vi "PCSMain.get Objects PCS-wide.vi"(0 "i ref in":refnum<vi>, 5 "error in (no error)":errorcluster) -> (14 "i ref out":refnum<vi>, 19 "error out":errorcluster)   [LabVIEW 2014, in "PCSMain.lvlib"]
doc: "This VI gets certain objects running elsewhere in the PCS."
uses:
  PCSMain.lvlib
  CS_Core/CSSystem/CSSystemLib/CSSystemLib.lvlib
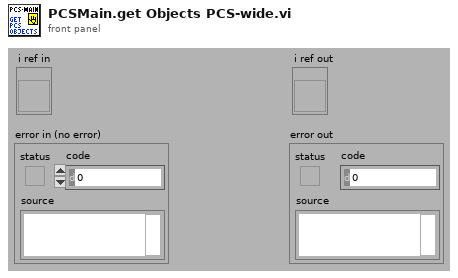
[diagram p1: front panel]
types:
  T1 = typedef "PCSMain.lvlib/PCSMain.i attribute.ctl" = cluster{"System Objects":cluster{"Spectrometer Objects":string[], "Camera Objects":string[], "Image Operator Objects":string[], "Gate- and Delaygenerators":string[], "Current Meas Objects":string[], "Calorimeter Objects":string[], "Powermeter Objects":string[], "SSAC Objects":string[], "Vacuum Control Objects":string[], "Countdown Counter Objects":string[], "Beckhoff Watchdog Objects":string[], "SHS Analyzer Objects":string[]}, "Local Objects":cluster{"Spectrometer Objects":string[], "Camera Objects":string[], "Image Operator Objects":string[], "Gate- and Delaygenerators":string[], "Current Meas Objects":string[], "Calorimeter Objects":string[], "Powermeter Objects":string[], "SSAC Objects":string[], "Vacuum Control Objects":string[], "Countdown Counter Objects":string[], "Beckhoff Watchdog Objects":string[], "SHS Analyzer Objects":string[]}, "Systems on same node":string[], "Data Viewer visible?":bool, "Running Objects":cluster{"Operators":bool, "SHS Analyzers":bool}, "Cam Instance System ID":string, "Black Box Objects":string[], "Switch Objects":string[], "Motion GUI Objects":string[], "Osci Objects":string[]}
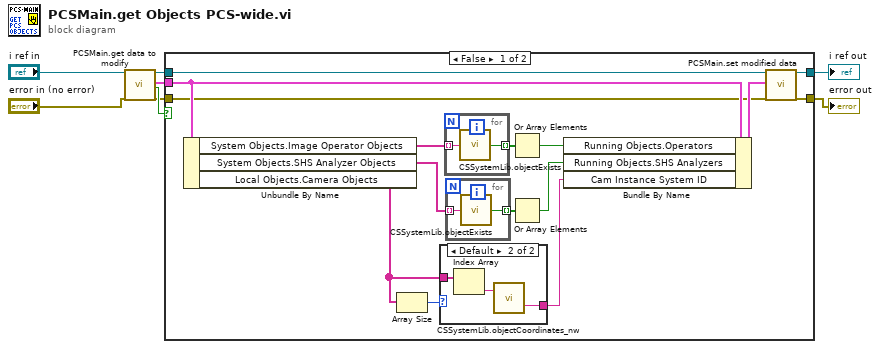
[diagram p0: block diagram]
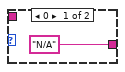
[diagram p2: hidden frame]
diagram:
  n1 = call "PCSMain.get data to modify.vi"("i ref in"="i ref in", "error in (no error)"="error in (no error)") -> ("i ref out"=w1:refnum<vi>, "i attribute"=w4:T1, "timed out"=w3:bool, "error out"=w2:errorcluster)  [unwired: 14 in]
  n2 = case shown="False" w3 {
    tunnel: w1 -> [w23 w33]
    tunnel: [w22 w33] -> w5
    tunnel: w2 -> [w18 w32]
    tunnel: [w21 w32] -> w6
    tunnel: w4 -> [w20 _]
    frame False {
      n3 = Unbundle By Name(w20) -> ("System Objects.Image Operator Objects"=w17:string[], "System Objects.SHS Analyzer Objects"=w14:string[], "Local Objects.Camera Objects"=w10:string[])
      n4 = Array Size(array=w10) -> (size(s)=w9:i32)
      n5 = case shown="Default" w9 {
        tunnel: w10 -> [_ w27]
        tunnel: ["N/A" ("systemID") w25] -> w11
        frame 0 {
        }
        frame Default {
          n6 = Index Array(array=w27) -> (element=w26:string)  [unwired: 1 in]
          n7 = call "CSSystemLib.objectCoordinates_nw.vi"("name"=w26) -> ("systemID"=w25:string)  [unwired: 15 in, 3 out]
        }
      }
      n8 = for {
        tunnel: w17 -> [w31] mode=indexing
        tunnel: [w30] -> w16 mode=indexing
        n9 = call "CSSystemLib.objectExists.vi"("name"=w31) -> ("obj exists"=w30:bool)
      }
      n10 = for {
        tunnel: w14 -> [w29] mode=indexing
        tunnel: [w28] -> w13 mode=indexing
        n11 = call "CSSystemLib.objectExists.vi"("name"=w29) -> ("obj exists"=w28:bool)
      }
      n12 = Or Array Elements(Boolean array=w16) -> (logical OR=w15:bool)
      n13 = Or Array Elements(Boolean array=w13) -> (logical OR=w12:bool)
      n14 = Bundle By Name(cluster=w20, "Running Objects.Operators"=w15, "Running Objects.SHS Analyzers"=w12, "Cam Instance System ID"=w11) -> (w19:T1)
      n15 = call "PCSMain.set modified data.vi"("i ref in"=w23, "i attribute"=w19, "error in (no error)"=w18) -> ("i ref out"=w22:refnum<vi>, "error out"=w21:errorcluster)  [unwired: 15 in]
    }
    frame True {
    }
  }
  "error out" <- w6
  "i ref out" <- w5
